vi "Get Event Data.vi"(6 "First T0":timestamp, 7 "CSV Settings":T1, 8 "Array Size":i32, 9 "group name":string, 10 "Header padding":string[](array[string]), 11 "Refnum in":refnum<k34>) -> (3 "Array out":string[][](array[string]))   [LabVIEW 2022 SP3, in "CSV Export.lvlib" / "CSV Export.lvclass"]
uses:
  CSV Export.lvclass
  Controls/CSV Export Settings.ctl
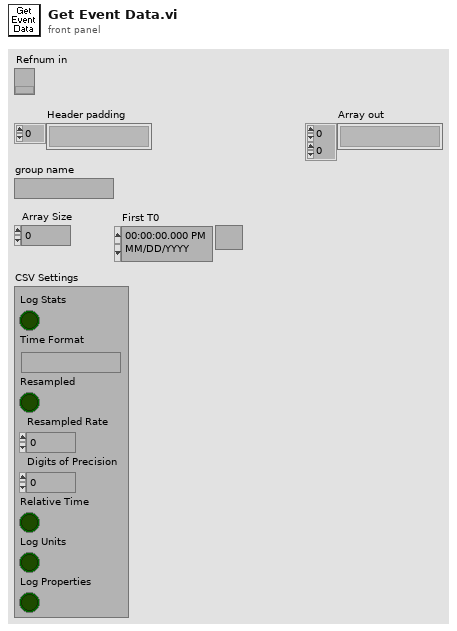
[diagram p1: front panel]
types:
  T1 = typedef "CSV Export.lvlib/CSV Export.lvclass/CSV Export Settings.ctl" = cluster{"Log Stats":bool, "Time Format":string, "Resampled":bool, "Resampled Rate":dbl, "Digits of Precision":u32, "Relative Time":bool, "Log Units":bool, "Log Properties":bool}
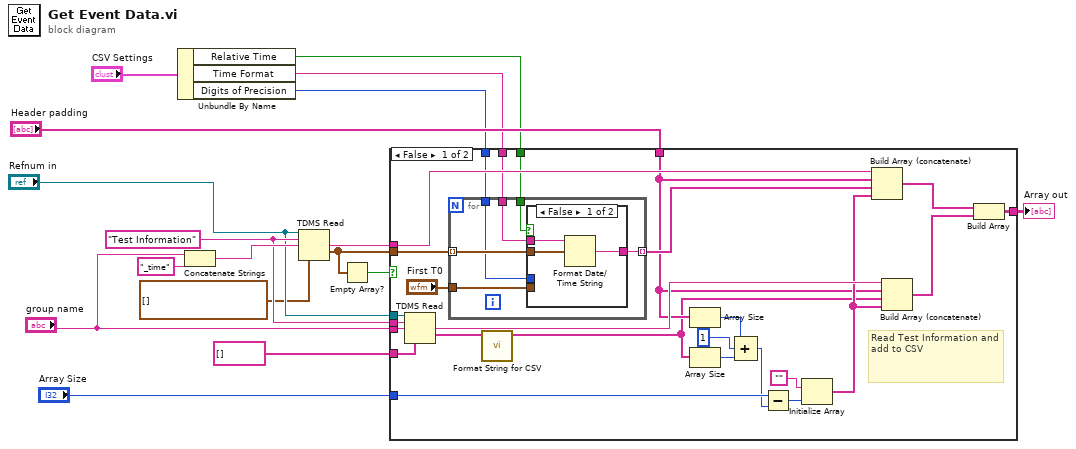
[diagram p0: block diagram]
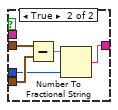
[diagram p2: hidden frame]
diagram:
  w12 = "Test Information" ("group name")
  n1 = Unbundle By Name("CSV Settings") -> ("Relative Time"=w4:bool, "Time Format"=w5:string, "Digits of Precision"=w3:u32)
  n2 = Concatenate Strings("group name", "_time" ("group name")) -> (w17:string)
  n3 = TDMS Read(0:"Refnum in", 5:w12, 7:w17, 12:timestamp[] []) -> (8:w9:string, 10:w2:timestamp[])  [unwired: 4 in, 4 out]
  n4 = Empty Array?(array=w2) -> (empty?=w1:bool)
  n5 = case shown="False" w1 {
    tunnel: "group name" -> [w43 _]
    tunnel: [w42 _] -> w14
    tunnel: string[] [] -> [w40 _]
    tunnel: w12 -> [w39 _]
    tunnel: "Refnum in" -> [w38 _]
    tunnel: "Array Size" -> [w36 _]
    tunnel: w9 -> [w33 _]
    tunnel: w2 -> [w32 _]
    tunnel: "Header padding" -> [w29 _]
    tunnel: w5 -> [w21 _]
    tunnel: w4 -> [w20 _]
    tunnel: w3 -> [w18 _]
    frame False {
      # "Read Test Information and add to CSV"
      n6 = TDMS Read(0:w38, 5:w39, 7:w43, 12:w40) -> (8:w41:string, 10:w25:string[])  [unwired: 4 in, 4 out]
      n7 = for {
        tunnel: w32 -> [w49] mode=indexing
        tunnel: [w48] -> w37 mode=indexing
        tunnel: w21 -> [w47]
        tunnel: w20 -> [w46]
        tunnel: "First T0" -> [w45]
        tunnel: w18 -> [w44]
        n8 = case shown="False" w46 {
          tunnel: w49 -> [w52 w57]
          tunnel: [w51 w54] -> w48
          tunnel: w47 -> [w50 _]
          tunnel: w45 -> [_ w56]
          tunnel: w44 -> [_ w53]
          frame False {
            n9 = Format Date/Time String(time format string (%c)=w50, seconds (now)=w52) -> (date/time string=w51:string)  [unwired: 1 in]
          }
          frame True {
            n10 = Subtract(x=w57, y=w56) -> (x-y=w55:dbl)
            n11 = Number To Fractional String(number=w55, precision (6)=w53) -> (F-format string=w54:string)  [unwired: 2 in]
          }
        }
      }
      n12 = call "Format String for CSV.vi"("Row Data"=w25) -> ("CSV Formatted strings"=w24:string[])  [unwired: 10 in]
      n13 = Array Size(array=w29) -> (size(s)=w28:i32)
      n14 = Array Size(array=w24) -> (size(s)=w30:i32)
      n15 = Compound Arithmetic op=ADD(w28, 1, w30) -> (w26:i32)
      n16 = Subtract(x=w36, y=w26) -> (x-y=w34:i32)
      n17 = Initialize Array("", w34) -> (w31:string[])
      n18 = Build Array (concatenate)(w33, w29, w37, w31) -> (w22:string[])
      n19 = Build Array (concatenate)(w41, w29, w24, w31) -> (w23:string[])
      n20 = Build Array(w22, w23) -> (w42:string[][])
    }
    frame True {
    }
  }
  "Array out" <- w14
